vi "_DServerReplyToReadAttribute.vi"(1 "attribute value":T1={"device name"="", "attribute name"="", "quality value"=0, "quality string"="", "timestamp"=0.0, "dim. x"=0, "dim. y"=0, "value"=[], "error code"=0, "error stack"=[], "data type"=36}, 2 "client request":T2={"Request Id"=0, "Source Id"=0, "Request Type"=enum."UNKNOWN_REQUEST", "Device Class Name"="unspecified/device/name", "Device Name"="unspecified_cmd_or_attr_name", "Cmd or Attr Name"="unspecified_cmd_or_attr_name", "Client Request Data"={"write attribute value"={"dimx"=0, "dimy"=0, "data"=[], "data_type"=enum."UNKNOWN_DATA_TYPE"}, "exec. command argin"={"num data"=[], "str data"=[]}}}, 3 "error in":errorcluster) -> (0 "error out":errorcluster)   [LabVIEW 2014, in "tango.lvlib"]
uses:
  tango.lvlib
  Client Request Handling/Typedefs/_DServerClientRequest.ctl
  Client Request Handling/Typedefs/_DServerClientRequestType.ctl
  Client Request Handling/Typedefs/_DServerClientRequestData.ctl
  Client Request Handling/Typedefs/_GenericDataBuffer.ctl
  Common VIs/Typedefs/_AttributeDataType_t.ctl
  tango_binding.so
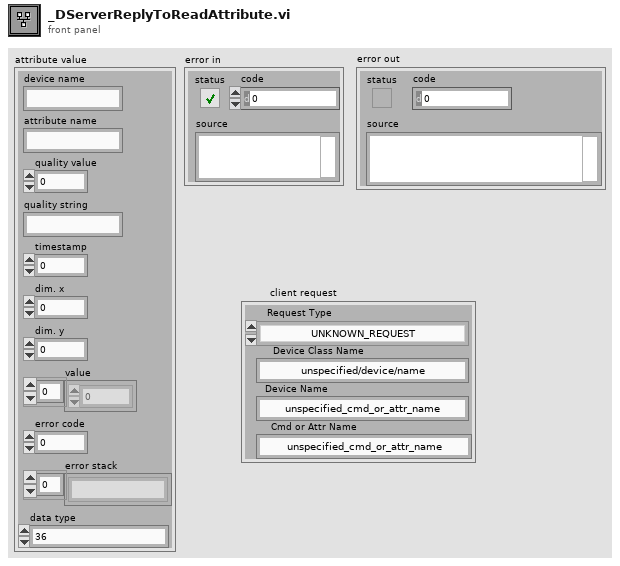
[diagram p1: front panel]
types:
  T1 = cluster{"device name":string, "attribute name":string, "quality value":i16, "quality string":string, "timestamp":dbl, "dim. x":i32, "dim. y":i32, "value":u8[], "error code":i32, "error stack":string[], "data type":u16}
  T2 = typedef "tango.lvlib/_DServerClientRequest.ctl" = cluster{"Request Id":u32, "Source Id":u32, "Request Type":T3, "Device Class Name":string, "Device Name":string, "Cmd or Attr Name":string, "Client Request Data":T4}
  T3 = typedef "tango.lvlib/_DServerClientRequestType.ctl" = enum16{"EXEC_CMD", "READ_ATTR", "WRITE_ATTR", "UNKNOWN_REQUEST"}
  T4 = typedef "tango.lvlib/_DServerClientRequestData.ctl" = cluster{"write attribute value":T5, "exec. command argin":cluster{"num data":u8[], "str data":string[]}}
  T5 = typedef "tango.lvlib/_GenericDataBuffer.ctl" = cluster{"dimx":u32, "dimy":u32, "data":u8[], "data_type":T6}
  T6 = typedef "tango.lvlib/_AttributeDataType_t.ctl" = enum16{"STATE_SCA", "STATE_SPE", "STATE_IMG", "STRING_SCA", "STRING_SPE", "STRING_IMG", "BOOL_SCA", "BOOL_SPE", "BOOL_IMG", "UCHAR_SCA", "UCHAR_SPE", "UCHAR_IMG", "SHORT_SCA", "SHORT_SPE", "SHORT_IMG", "USHORT_SCA", "USHORT_SPE", "USHORT_IMG", "LONG_SCA", "LONG_SPE", "LONG_IMG", "ULONG_SCA", "ULONG_SPE", "ULONG_IMG", "LONG64_SCA", "LONG64_SPE", "LONG64_IMG", "ULONG64_SCA", "ULONG64_SPE", "ULONG64_IMG", "FLOAT_SCA", "FLOAT_SPE", "FLOAT_IMG", "DOUBLE_SCA", "DOUBLE_SPE", "DOUBLE_IMG", "ENUM_SCA", "UNKNOWN_DATA_TYPE"}
  T7 = cluster{"Request Id":u32, "Source Id":u32, u32, "error stack":string[]}
  T8 = cluster{cluster{"Request Id":u32, "Source Id":u32, u32, "error stack":string[]}, "attribute value":cluster{"device name":string, "attribute name":string, "quality value":i16, "quality string":string, "timestamp":dbl, "dim. x":i32, "dim. y":i32, "value":u8[], "error code":i32, "error stack":string[], "data type":u16}}
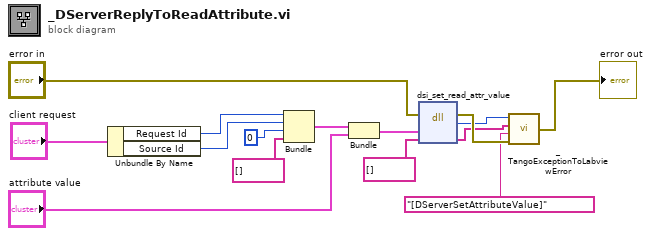
[diagram p0: block diagram]
diagram:
  n1 = Unbundle By Name("client request") -> ("Request Id"=w7:u32, "Source Id"=w6:u32)
  n2 = Bundle("Request Id"=w7, "Source Id"=w6, u32 0, "error stack"=string[] []) -> (w3:T7)  [unwired: 1 in]
  n3 = Bundle(w3, "attribute value"="attribute value") -> (w2:T8)  [unwired: 1 in]
  n4 = dll-call lib="tango_binding.*" fn="dsi_set_read_attr_value"(error in="error in", "attribute_value"=w2, "error_stack"=string[] [] ("error stack")) -> (error out=w12:errorcluster, "return type"=w10:i32, "error_stack"=w11:string[])  [unwired: 3 in, 1 out]
  n5 = call "_TangoExceptionToLabviewError.vi"("error in"=w12, "location"="[DServerSetAttributeValue]", "error stack"=w11, "error code"=w10) -> ("error out"=→"error out":errorcluster)
